vi "save-one-image-in-file.vi"() -> ()   [LabVIEW 2011, in "librir.lvlib"]
uses:
  librir.lvlib
panel:
  out "error out":errorcluster
  in  "filename":path=path "d:/Users/CEA/Desktop/a.h264"
  in  "img":u16[][](array[numeric])=array515x640[329600 elements]
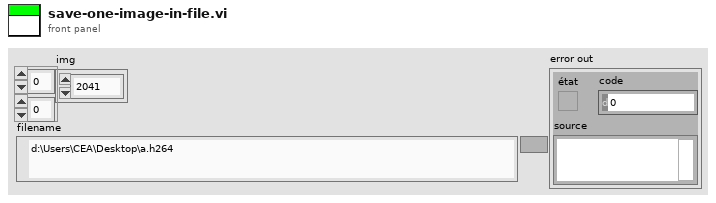
[diagram p1: front panel]
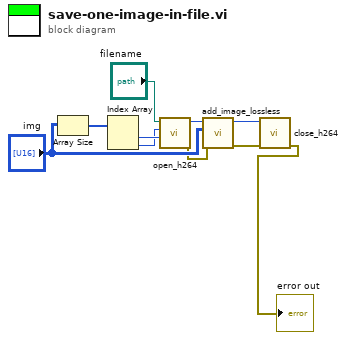
[diagram p0: block diagram]
diagram:
  n1 = Array Size(array="img") -> (size(s)=w6:i32[])
  n2 = Index Array(array=w6) -> (element #1=w5:i32, element #2=w4:i32)  [unwired: 2 in]
  n3 = call "open_h264.vi"("height"=w5, "width"=w4, "filename"="filename") -> ("error out"=w3:errorcluster, "h264_file_handle"=w10:u64)  [unwired: 7 in]
  n4 = call "add_image_lossless.vi"("error in (no error)"=w3, "img"="img", "h264_file_handle"=w10) -> ("error out"=w2:errorcluster, "h264_file_handle"=w9:u64)  [unwired: 7 in]
  n5 = call "close_h264.vi"("error in (no error)"=w2, "ir_file_handler"=w9) -> ("error out"=→"error out":errorcluster)  [unwired: 8 in, 1 out]
